vi "PH_AWG-510.PC Get Output Settings.vi"(0 "VI in":refnum<vi>, 5 "error in (no error)":errorcluster) -> (14 "VI out":refnum<vi>, 19 "error out":errorcluster)   [LabVIEW 2014, in "PH_AWG-510.lvlib"]
doc: "This VI requests the current output settings to store them at own attributes and to tisplay them at the GUI."
uses:
  PH_AWG-510.lvlib
  instr.lib/awg510/Tektronix AWG510.lvlib
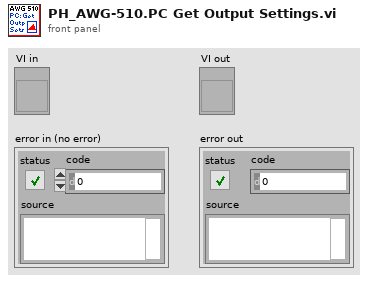
[diagram p1: front panel]
types:
  T1 = typedef "PH_AWG-510.lvlib/PH_AWG-510.i attribute.ctl" = cluster{"GUI Refs":cluster{"Delete":refnum<vi>, "Trigger Settings":refnum<vi>, "Start Device":refnum<vi>, "Instrument Information":refnum<vi>, "Lock Frontpanel":refnum<vi>, "Waveform Pattern File":refnum<vi>, "Initialize":refnum<vi>, "Output Settings":refnum<vi>}, "Instrument Information":T2, "Initialized?":bool, "Current Settings":cluster{"Trigger":T3, "Output Settings":T4}, "Wanted Settings":cluster{"Trigger":T3, "Output Settings":T4}, "Device frontpanel locked?":bool, "Default File Path":path}
  T2 = typedef "PH_AWG-510.lvlib/PH_AWG-510.Instrument Information Dataset.ctl" = cluster{"VISA resource name":refnum<visa-resource-name>, "Instrument Firmware Revision":string, "Manufacturer":string, "Model":string, "Serial Number":string, "Error Message":string, "Device Status":enum16{"stopped", "wating for trigger", "running", "Failure"}}
  T3 = typedef "PH_AWG-510.lvlib/PH_AWG-510.Trigger Settings.ctl" = cluster{"Mode":enum16{"Continuous", "Triggered", "Gated", "Enhanced"}, "Level (V)":dbl, "External Source":bool}
  T4 = typedef "PH_AWG-510.lvlib/PH_AWG-510.Output Settings.ctl" = cluster{"Activate Channel":bool, "VPP (V)":dbl, "Clock (Hz)":dbl, "File Name (Device)":string, "#1":u16, "#2":u16, "#3":u16, "#4":u16, "#5":u16, "#6":u16, "#7":u16, "#8":u16, "#9":u16, "#10":u16, "#11":u16, "#12":u16, "#13":u16, "#14":u16, "#15":u16, "#16":u16, "#17":u16, "#18":u16, "#19":u16, "#20":u16, "Offset (V)":dbl}
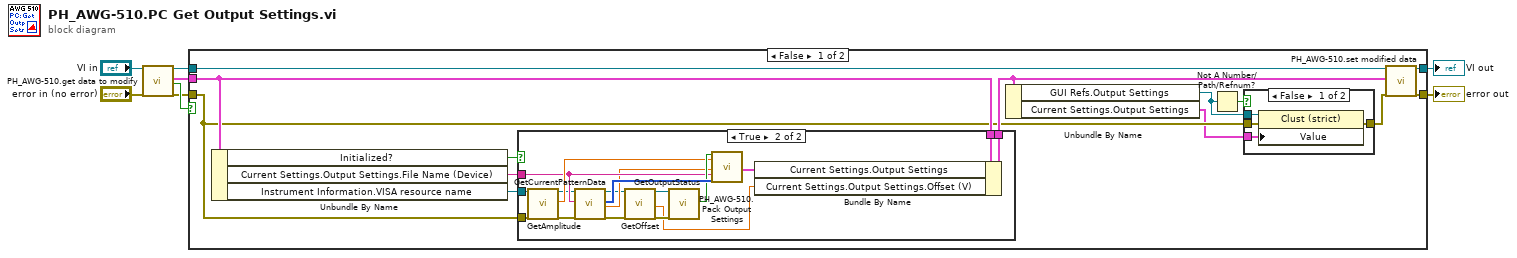
[diagram p0: block diagram]
diagram:
  n1 = call "PH_AWG-510.get data to modify.vi"("i ref in"="VI in", "error in (no error)"="error in (no error)") -> ("i ref out"=w6:refnum<vi>, "i attribute"=w7:T1, "timed out"=w8:bool, "error out"=w4:errorcluster)  [unwired: 14 in]
  n2 = case shown="False" w8 {
    tunnel: w4 -> [w11 w46]
    tunnel: [w21 w46] -> w2
    tunnel: w6 -> [w20 w45]
    tunnel: w7 -> [w18 _]
    tunnel: [w19 w45] -> w1
    frame False {
      n3 = Unbundle By Name(w18) -> ("Initialized?"=w16:bool, "Current Settings.Output Settings.File Name (Device)"=w13:string, "Instrument Information.VISA resource name"=w17:refnum<visa-resource-name>)
      n4 = case shown="True" w16 {
        tunnel: [w27 w44] -> w14
        tunnel: w18 -> [w27 w43]
        tunnel: w17 -> [_ w41]
        tunnel: w11 -> [_ w42]
        tunnel: w13 -> [_ w36]
        frame False {
        }
        frame True {
          n5 = call "GetAmplitude.vi"("VISA resource name"=w41, "error in"=w42) -> ("VISA resource name out"=w33:refnum<visa-resource-name>, "Amplitude (V)"=w37:dbl, "error out"=w32:errorcluster)  [unwired: 15 in]
          n6 = call "GetCurrentPatternData.vi"("VISA resource name"=w33, "File Name (xy.pat)"=w36, "error in"=w32) -> ("VISA resource name out"=w30:refnum<visa-resource-name>, "waveform array"=w39:u16[], "clock (Hz)"=w35:dbl, "error out"=w40:errorcluster)  [unwired: 13 in]
          n7 = call "GetOffset.vi"("VISA resource name"=w30, "error in"=w40) -> ("VISA resource name out"=w29:refnum<visa-resource-name>, "Offset (V)"=w28:dbl, "error out"=w31:errorcluster)  [unwired: 15 in]
          n8 = call "GetOutputStatus.vi"("VISA resource name"=w29, "error in"=w31) -> ("Output Status"=w38:bool)  [unwired: 15 in, 2 out]
          n9 = call "PH_AWG-510.Pack Output Settings.vi"("Activate Channel"=w38, "VPP [Volts]"=w37, "Clock [Hz]"=w35, "File Name"=w36, "Waveform Pattern [#1 ... #20]"=w39) -> ("Output Settings"=w34:T4)  [unwired: 14 in]
          n10 = Bundle By Name(cluster=w43, "Current Settings.Output Settings"=w34, "Current Settings.Output Settings.Offset (V)"=w28) -> (w44:T1)
        }
      }
      n11 = Unbundle By Name(w14) -> ("GUI Refs.Output Settings"=w12:refnum<vi>, "Current Settings.Output Settings"=w10:T4)
      n12 = Not A Number/Path/Refnum?(number/path/refnum=w12) -> (NaN/Path/Refnum?=w15:bool)
      n13 = case shown="False" w15 {
        tunnel: w11 -> [w25 w26]
        tunnel: [w24 w26] -> w9
        tunnel: w12 -> [w23 _]
        tunnel: w10 -> [w22 _]
        frame False {
          n14 = property class="Clust (strict)"(reference=w23, error in=w25, "Value"=w22) -> (error out=w24:errorcluster)  [unwired: 1 out]
        }
        frame True {
        }
      }
      n15 = call "PH_AWG-510.set modified data.vi"("i ref in"=w20, "i attribute"=w14, "error in (no error)"=w9) -> ("i ref out"=w19:refnum<vi>, "error out"=w21:errorcluster)  [unwired: 15 in]
    }
    frame True {
    }
  }
  "VI out" <- w1
  "error out" <- w2
